vi "Teste.vi"() -> ()   [LabVIEW 2020]
uses:
  C:/Users/Opto/Downloads/GrabTestTDNI/GrabFrame4.dll
  Downloads/GrabTestTDNI/GrabFrame4.dll
  C:/Users/Opto/Desktop/Equipamentos/Teste/DALSA.SaperaLT.SapClassBasic.dll
  DALSA.SaperaLT.SapClassBasic.dll
panel:
  in  "número de frames:":i32=3
  out "error SaveFrame":errorcluster
  out "error final":errorcluster
  out "error sapTransfer Dispose":errorcluster
  out "countFrame":i32
  out "Wait":bool
  out "Destroy":bool
  out "Create":bool
  out "framesArr":i16[][](array[numeric])
  out "Abriu arquivo?":bool
  out "filePath":string="C:\\temp\\IC-47_TDI.ccf"
  # "Buffer"
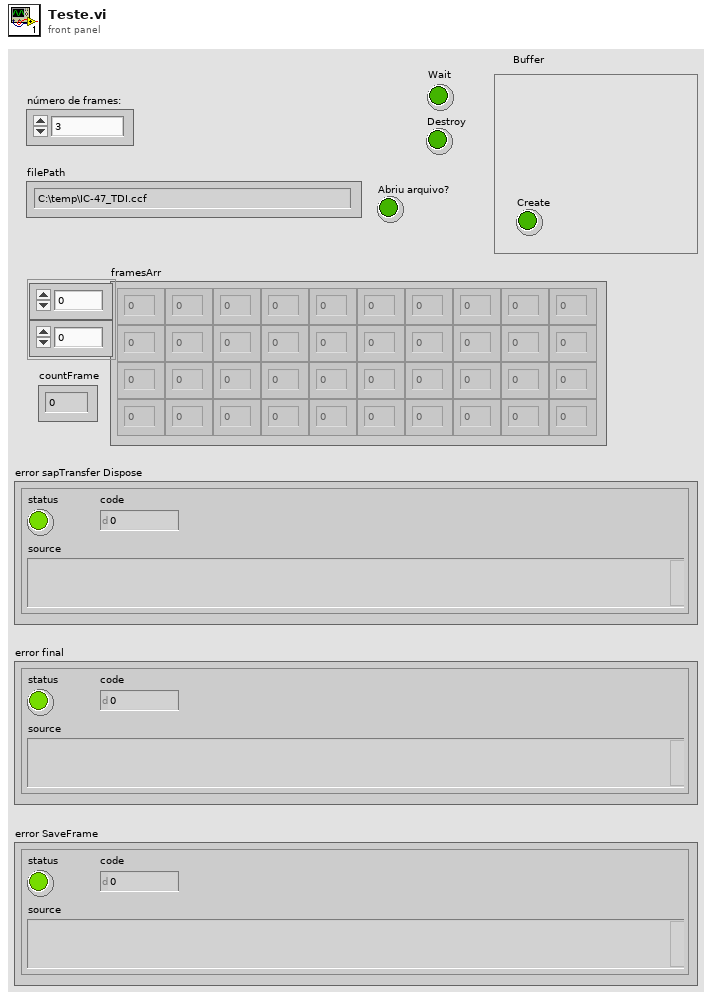
[diagram p1: front panel]
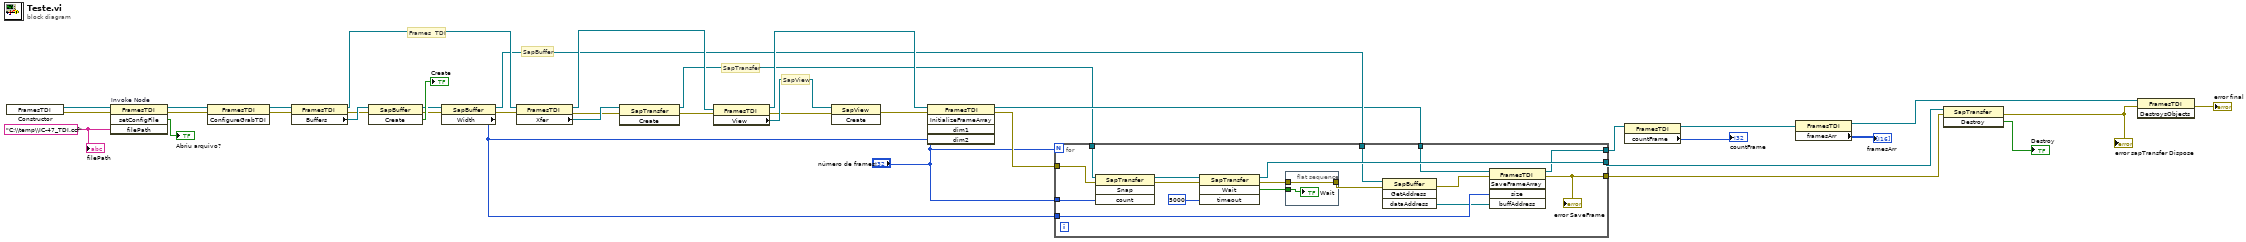
[diagram p0: block diagram]
diagram:
  w35 = "C:\\temp\\IC-47_TDI.ccf" ("filePath")
  # "SapView"
  # "SapTransfer"
  # "SapBuffer"
  # "Frames  TDI"
  n1 = constructor class="FramesTDI"() -> (reference out=w38:refnum<k24>, error out=w39:errorcluster)  [unwired: 3 in, 1 out]
  n2 = invoke on="Invoke Node" class="FramesTDI" method="setConfigFile"(reference=w38, error in=w39, "filePath"=w35) -> (reference out=w37:refnum<k24>, error out=w36:errorcluster, "setConfigFile"=→"Abriu arquivo?":bool)  [unwired: 1 in, 1 out]
  n3 = invoke class="FramesTDI" method="ConfigureGrabTDI"(reference=w37, error in=w36) -> (reference out=w33:refnum<k24>, error out=w27:errorcluster)  [unwired: 1 in, 1 out]
  n4 = property class="FramesTDI"(reference=w33, error in=w27) -> (reference out=w20:refnum<k24>, error out=w26:errorcluster, "Buffers"=w32:refnum<k24>)
  n5 = invoke class="SapBuffer" method="Create"(reference=w32, error in=w26) -> (reference out=w28:refnum<k24>, error out=w25:errorcluster, "Create"=→"Create":bool)  [unwired: 1 in]
  n6 = property class="SapBuffer"(reference=w28, error in=w25) -> (reference out=w12:refnum<k24>, error out=w24:errorcluster, "Width"=w10:i32)
  n7 = property class="FramesTDI"(reference=w20, error in=w24) -> (reference out=w18:refnum<k24>, error out=w23:errorcluster, "Xfer"=w31:refnum<k24>)
  n8 = invoke class="SapTransfer" method="Create"(reference=w31, error in=w23) -> (reference out=w5:refnum<k24>, error out=w22:errorcluster)  [unwired: 1 in, 1 out]
  n9 = property class="FramesTDI"(reference=w18, error in=w22) -> (reference out=w17:refnum<k24>, error out=w21:errorcluster, "View"=w30:refnum<k24>)
  n10 = invoke class="SapView" method="Create"(reference=w30, error in=w21) -> (error out=w19:errorcluster)  [unwired: 1 in, 2 out]
  n11 = invoke class="FramesTDI" method="InitializeFrameArray"(reference=w17, error in=w19, "dim1"="número de frames:", "dim2"=w10) -> (reference out=w11:refnum<k24>, error out=w14:errorcluster)  [unwired: 1 in, 3 out]
  n12 = for {
    N: "número de frames:" -> [_]
    tunnel: w5 -> [w56]
    tunnel: w14 -> [w55]
    tunnel: "número de frames:" -> [w54]
    tunnel: [w51] -> w13
    tunnel: w12 -> [w47]
    tunnel: w11 -> [w45]
    tunnel: w10 -> [w43]
    tunnel: [w41] -> w7
    tunnel: [w40] -> w9
    n13 = invoke class="SapTransfer" method="Snap"(reference=w56, error in=w55, "count"=w54) -> (reference out=w53:refnum<k24>, error out=w52:errorcluster)  [unwired: 1 in, 2 out]
    n14 = invoke class="SapTransfer" method="Wait"(reference=w53, error in=w52, "timeout"=5000) -> (reference out=w51:refnum<k24>, error out=w48:errorcluster, "Wait"=w49:bool)  [unwired: 1 in, 1 out]
    n15 = flat-sequence {
      tunnel: w49 -> [w58]
      tunnel: w48 -> [w57]
      tunnel: [w57] -> w46
      frame #0 {
        "Wait" <- w58
      }
    }
    n16 = invoke class="SapBuffer" method="GetAddress"(reference=w47, error in=w46) -> (error out=w44:errorcluster, "dataAddress"=w42:refnum<k24>)  [unwired: 2 in, 2 out]
    n17 = invoke class="FramesTDI" method="SaveFrameArray"(reference=w45, error in=w44, "size"=w43, "buffAddress"=w42) -> (reference out=w41:refnum<k24>, error out=w40:errorcluster)  [unwired: 1 in, 3 out]
    "error SaveFrame" <- w40
  }
  n18 = property class="FramesTDI"(reference=w7) -> (reference out=w8:refnum<k24>, "countFrame"=→"countFrame":i32)  [unwired: 1 in, 1 out]
  n19 = property class="FramesTDI"(reference=w8) -> (reference out=w4:refnum<k24>, "framesArr"=→"framesArr":i16[][])  [unwired: 1 in, 1 out]
  n20 = invoke class="SapTransfer" method="Destroy"(reference=w13, error in=w9) -> (error out=w2:errorcluster, "Destroy"=→"Destroy":bool)  [unwired: 1 in, 1 out]
  "error sapTransfer Dispose" <- w2
  n21 = invoke class="FramesTDI" method="DestroysObjects"(reference=w4, error in=w2) -> (error out=→"error final":errorcluster)  [unwired: 1 in, 2 out]
  "filePath" <- w35
